vi "LLB Pre-Build CHM Build.vi"(6 "Top Level/Always Included VIs":path[](array[path]), 7 "Main Destination Path":path, 9 "Target Name":string, 10 "Build Specification Name":string, 11 "Project Path":path) -> (0 "error out":errorcluster)   [LabVIEW 2024]
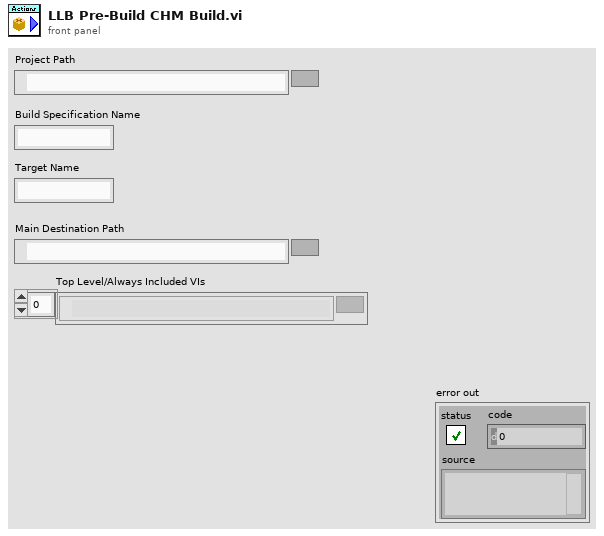
[diagram p1: front panel]
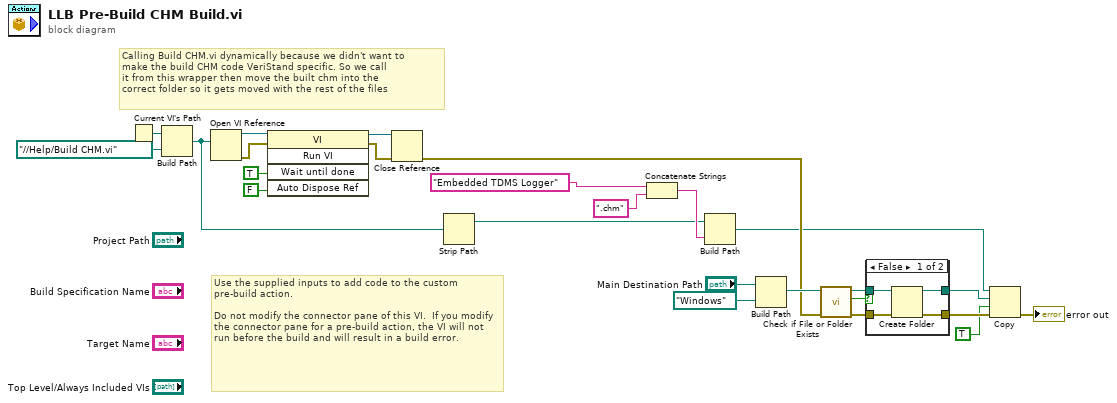
[diagram p0: block diagram]
diagram:
  # "Calling Build CHM.vi dynamically because we didn't want to \nmake the build CHM code VeriStand specific. So we call\nit from this wrapper then move the built chm into the\ncorrect folder so it gets moved with the rest of the files"
  # "Use the supplied inputs to add code to the custom pre-build action.\n\nDo not modify the connector pane of this VI.  If you modify the connector pane for a pre-build action, the VI will not run before the build and will result in a build error."
  n1 = Current VI's Path() -> (path=w25:path)
  n2 = Build Path(base path=w25, name or relative path=path "../../Help/Build CHM.vi") -> (appended path=w17:path)
  n3 = Open VI Reference(vi path=w17) -> (vi reference=w23:refnum<vi>, error out=w22:errorcluster)  [unwired: 5 in]
  n4 = invoke class="VI" method="Run VI"(reference=w23, error in=w22, "Wait until done"=TRUE ("Wait Until Done"), "Auto Dispose Ref"=FALSE ("Auto Dispose Reference")) -> (reference out=w19:refnum<vi>, error out=w18:errorcluster)  [unwired: 1 in, 3 out]
  n5 = Close Reference(reference=w19, error in (no error)=w18) -> (error out=w11:errorcluster)
  n6 = Strip Path(path=w17) -> (stripped path=w2:path)  [unwired: 1 out]
  n7 = Concatenate Strings("Embedded TDMS Logger" ("string"), ".chm" ("string")) -> (w15:string)
  n8 = Build Path(base path=w2, name or relative path=w15) -> (appended path=w4:path)
  n9 = Build Path(base path="Main Destination Path", name or relative path=path "Windows") -> (appended path=w12:path)
  n10 = call <vilib>:"Check if File or Folder Exists.vi"("error in (no error)"=w11, "path"=w12) -> ("error out"=w8:errorcluster, "file or folder exists?"=w10:bool, "dup path"=w9:path)  [unwired: 7 in]
  n11 = case shown="False" w10 {
    tunnel: w9 -> [w28 w31]
    tunnel: w8 -> [w29 w30]
    tunnel: [w27 w31] -> w6
    tunnel: [w26 w30] -> w7
    frame False {
      n12 = Create Folder(path (use dialog)=w28, error in=w29) -> (created path=w27:path, error out=w26:errorcluster)  [unwired: 1 in, 1 out]
    }
    frame True {
    }
  }
  n13 = Copy(8:w7, 9:TRUE ("overwrite (F)"), 10:w6, 11:w4) -> (0:→"error out":errorcluster)  [unwired: 1 in, 2 out]
